vi "Start Trigger Simple Analog Channel.vi"(6 "Event types (Edge or Level)":u16(ring) items=["Edge", "Level"], 8 "error in (no error)":errorcluster, 10 "Trigger consign":T1 {"Channel" items=["A1"=0, "A2"=1, "A3"=2, "A4"=3, "A5"=4, "A6"=5, "A7"=6, "A8"=7, "A9"=8, "A10"=9, "K1"=200, "K2"=201, "K3"=202, "K4"=203, "FA1"=204, "FA2"=205, "FA3"=206, "FA4"=207]; "Assign to S1 or S2 threshold?" items=["S1", "S2"]; "Positive or negative (edge or level)" items=["Positive", "Negative"]}, 11 "VISA resource name":refnum<visa-resource-name>) -> (0 "error out":errorcluster, 3 "VISA resource name out":refnum<visa-resource-name>)   [LabVIEW 2017, in "Sefram DAS220.lvlib"]
doc: "Start recording on an event on a simple channel. For example, if A1 channel raised 4V."
uses:
  <instrlib>/Sefram DAS220/Sefram DAS220.lvlib
  <instrlib>/Sefram DAS220/Public/Configure/Triggers-Alarms/Low-level/Trigger Types/Complex Trigger Consign.ctl
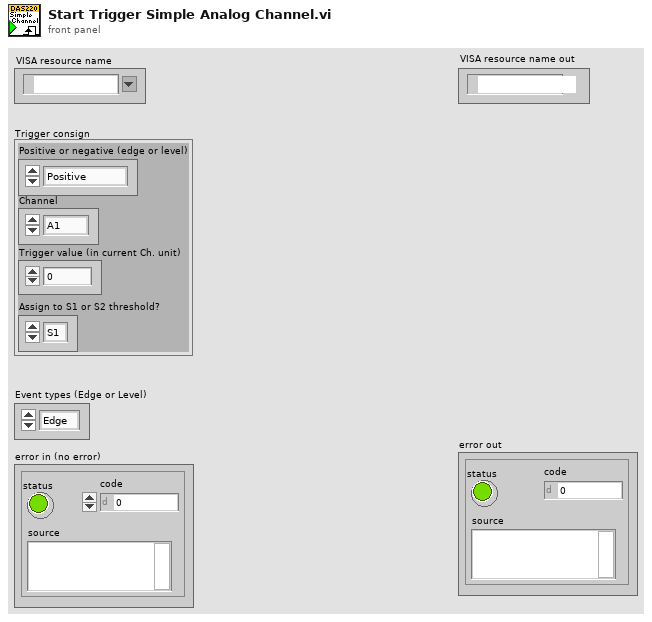
[diagram p1: front panel]
types:
  T1 = typedef "Sefram DAS220.lvlib/Complex Trigger Consign.ctl" = cluster{"Trigger value (in current Ch. unit)":dbl, "Positive or negative (edge or level)":u16, "Assign to S1 or S2 threshold?":u16, "Channel":u16}
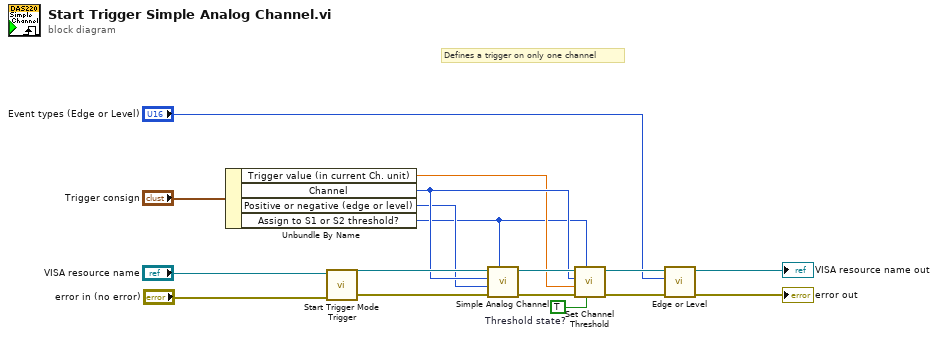
[diagram p0: block diagram]
diagram:
  w3 = TRUE  # Threshold state?
  # "Defines a trigger on only one channel"
  n1 = Unbundle By Name("Trigger consign") -> ("Trigger value (in current Ch. unit)"=w5:dbl, "Channel"=w6:u16, "Positive or negative (edge or level)"=w4:u16, "Assign to S1 or S2 threshold?"=w2:u16)
  n2 = call <instrlib>:"Start Trigger Mode Trigger.vi"("error in (no error)"="error in (no error)", "VISA resource name"="VISA resource name") -> ("error out"=w9:errorcluster, "VISA resource name out"=w8:refnum<visa-resource-name>)  [unwired: 8 in]
  n3 = call <instrlib>:"Simple Analog Channel.vi"("S1 or S2"=w2, "error in (no error)"=w9, "Positive or negative (edge or level)"=w4, "Channel"=w6, "VISA resource name"=w8) -> ("error out"=w10:errorcluster, "VISA resource name out"=w11:refnum<visa-resource-name>)  [unwired: 5 in]
  n4 = call <instrlib>:"Set Channel Threshold.vi"("Threshold state?"=w3, "Threshold S1/S2"=w2, "error in (no error)"=w10, "Threshold value (in actual channel unit)"=w5, "Channel"=w6, "VISA resource name"=w11) -> ("error out"=w14:errorcluster, "VISA resource name out"=w15:refnum<visa-resource-name>)  [unwired: 4 in]
  n5 = call <instrlib>:"Edge or Level.vi"("error in (no error)"=w14, "Event types (Edge or Level)"="Event types (Edge or Level)", "VISA resource name"=w15) -> ("error out"=→"error out":errorcluster, "VISA resource name out"=→"VISA resource name out":refnum<visa-resource-name>)  [unwired: 7 in]
